vi "worksheet set background buffer.vi"(8 "error in (no error)":errorcluster, 9 "image_size":u32, 10 "image_buffer":string, 11 "worksheet":u32) -> (0 "error out":errorcluster, 3 "function return":u32(ring))   [LabVIEW 8.6]
doc: "lxw_error worksheet_set_background_buffer(lxw_worksheet worksheet, const unsigned char *image_buffer, size_t image_size);"
uses:
  pending_lvxlsxwriter/xlsxwriter.dll
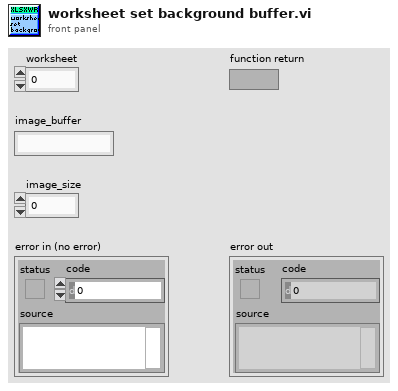
[diagram p1: front panel]
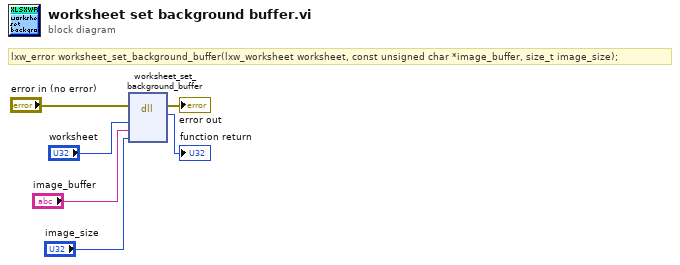
[diagram p0: block diagram]
diagram:
  # "lxw_error worksheet_set_background_buffer(lxw_worksheet worksheet, const unsigned char *image_buffer, size_t image_size);"
  n1 = dll-call lib="C:/Users/WDAGUtilityAccount/Desktop/pending_lvxlsxwriter/xlsxwriter.*" fn="worksheet_set_background_buffer"(error in="error in (no error)", "worksheet"="worksheet", "image_buffer"="image_buffer", "image_size"="image_size") -> (error out=→"error out":errorcluster, →"function return":u32)  [unwired: 5 in, 1 out]
